vi "压装试验判定.vi"(7 "Result":refnum<vi>, 10 "判定参数":T1, 11 "XY曲线":cluster{"X":dbl[], "Y":dbl[]}[](array[cluster])) -> (2 "判定项长度":i32, 3 "OK？":bool)   [LabVIEW 2020]
panel:
  out "上限":dbl
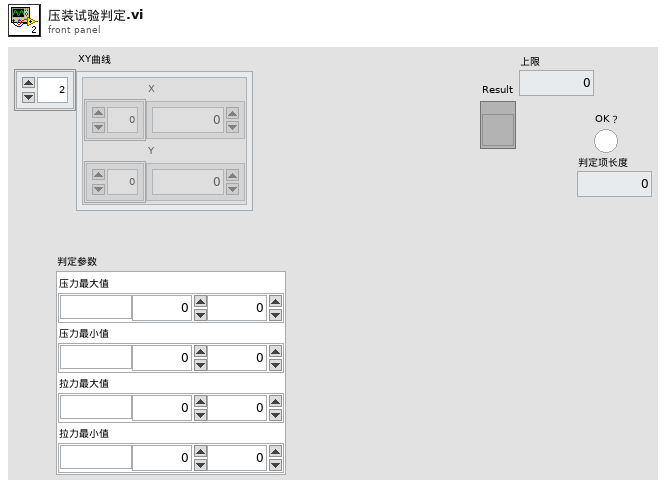
[diagram p1: front panel]
types:
  T1 = cluster{"压力最大值":cluster{"单位":string, "下限":dbl, "上限":dbl}, "压力最小值":cluster{"单位":string, "下限":dbl, "上限":dbl}, "拉力最大值":cluster{"单位":string, "下限":dbl, "上限":dbl}, "拉力最小值":cluster{"单位":string, "下限":dbl, "上限":dbl}}
  T2 = cluster{"位移":cluster{"单位":string, "下限":dbl, "上限":dbl}, "压力":cluster{"单位":string, "下限":dbl, "上限":dbl}}
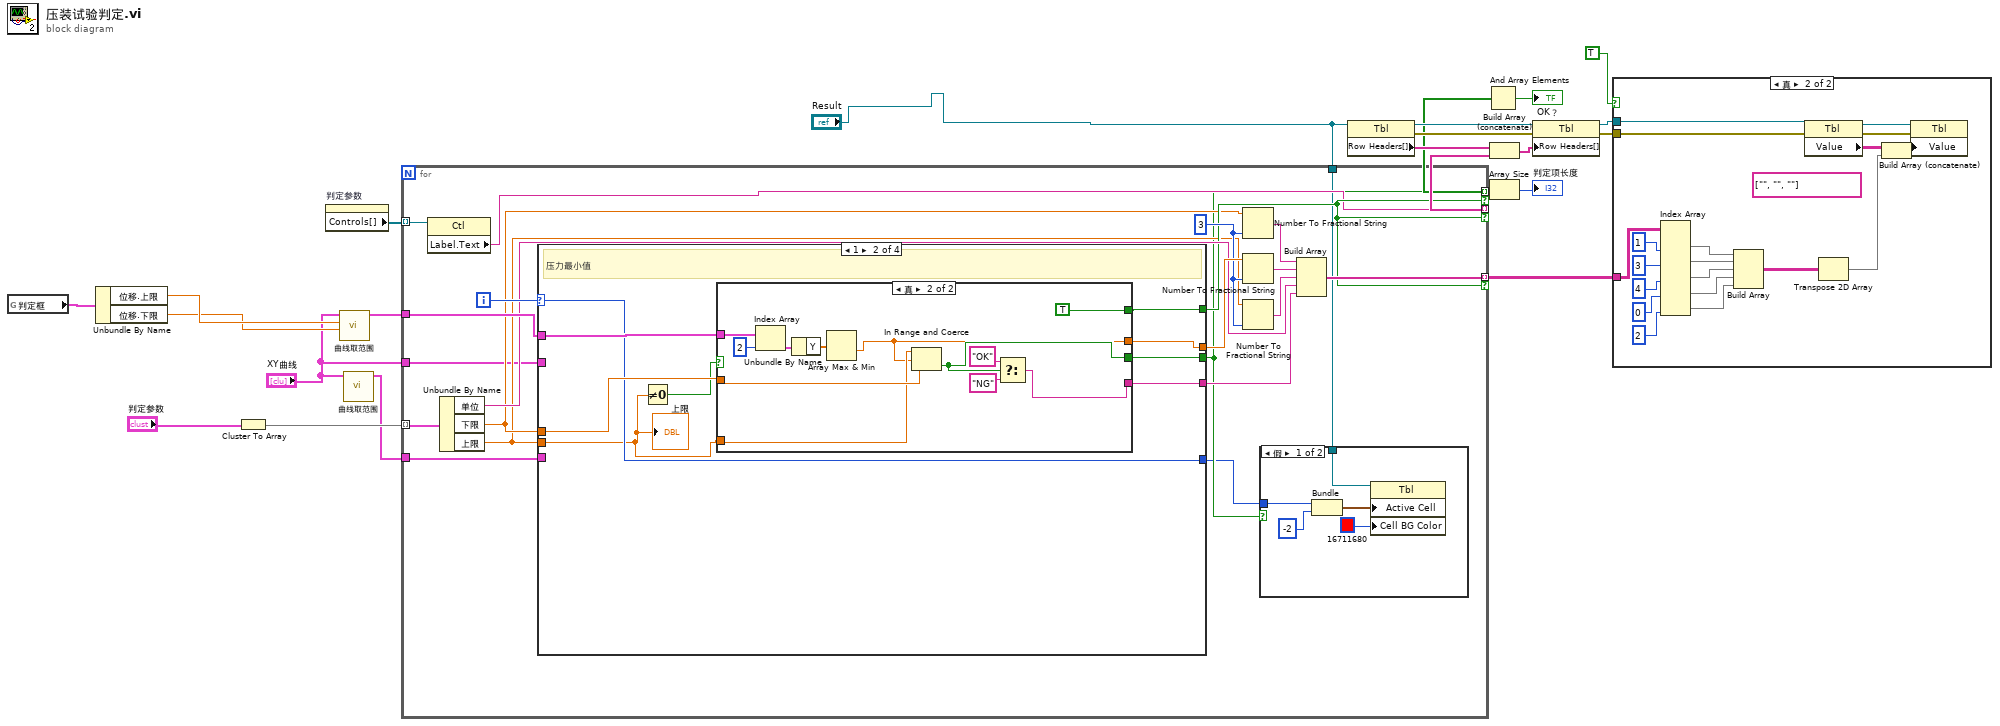
[diagram p0: block diagram]
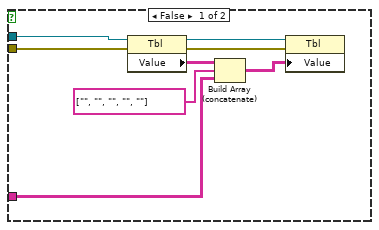
[diagram p2: hidden frame]
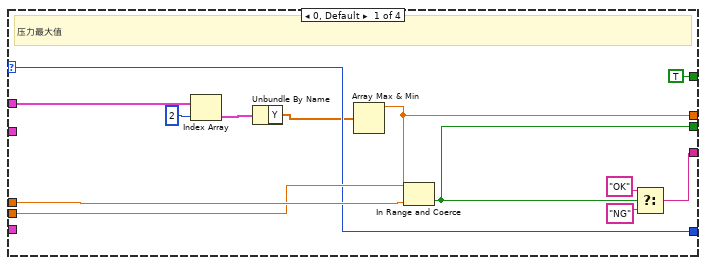
[diagram p4: hidden frame]
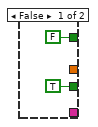
[diagram p5: hidden frame]
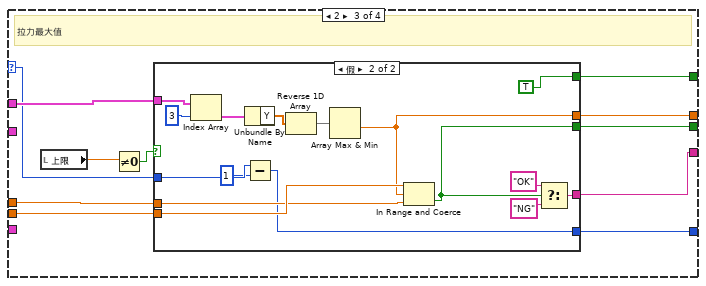
[diagram p6: hidden frame]
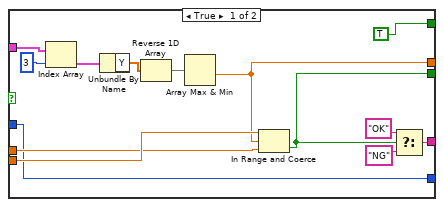
[diagram p7: hidden frame]
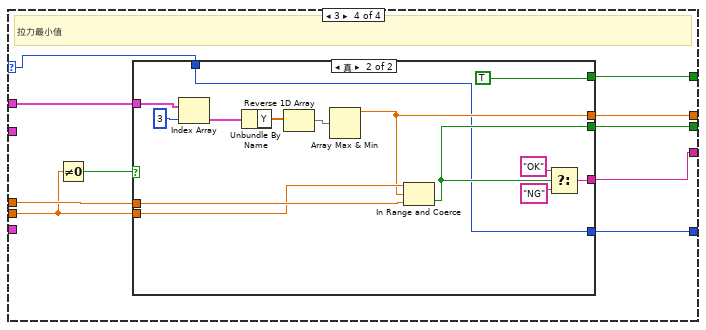
[diagram p8: hidden frame]
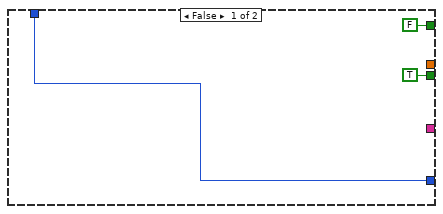
[diagram p9: hidden frame]
diagram:
  n1 = global read "判定参数.vi" "判定框"() -> (w4:T2)
  n2 = Unbundle By Name(w4) -> ("位移.上限"=w6:dbl, "位移.下限"=w5:dbl)
  n3 = Cluster To Array(cluster="判定参数") -> (array=w22:cluster{"单位":string, "下限":dbl, "上限":dbl}[])
  n4 = property on="判定参数" class="Clust (严格)"() -> ("Controls[]"=w12:refnum<vi>[])  [unwired: 2 in, 2 out]
  n5 = call "曲线取范围.vi"("下限"=w5, "上限"=w6, "曲线In"="XY曲线") -> ("曲线Out"=w8:cluster{"X":dbl[], "Y":dbl[]}[])  [unwired: 8 in]
  n6 = call "曲线取范围.vi"("曲线In"="XY曲线") -> ("曲线Out"=w2:cluster{"X":dbl[], "Y":dbl[]}[])  [unwired: 10 in]
  n7 = for {
    tunnel: w22 -> [w43] mode=indexing
    tunnel: w12 -> [w41] mode=indexing
    tunnel: w8 -> [w39]
    tunnel: [w24] -> w10 mode=indexing if=w31
    tunnel: [w32] -> w13 mode=indexing if=w31
    tunnel: [w28] -> w15 mode=indexing if=w31
    tunnel: "XY曲线" -> [w27]
    tunnel: w2 -> [w26]
    tunnel: "Result" -> [w25]
    i -> [w42]
    w38 = i16 3 ("精度(6)")
    n8 = property class="Ctl"(reference=w41) -> ("Label.Text"=w28:string)  [unwired: 1 in, 2 out]
    n9 = Unbundle By Name(w43) -> ("单位"=w33:string, "下限"=w30:dbl, "上限"=w29:dbl)
    n10 = case shown="1" w42 {
      selector: w42 -> [w51 w65 w86 w127]
      tunnel: [w49 w64 w92 w132] -> w40
      tunnel: w39 -> [w61 w70 w91 w131]
      tunnel: [w56 w69 w95 w135] -> w34
      tunnel: [w55 w68 w94 w134] -> w24
      tunnel: w30 -> [w54 w67 w90 w130]
      tunnel: w29 -> [w53 w62 w93 w128]
      tunnel: [TRUE w66 w89 w133] -> w31
      tunnel: w27 -> [_ _ _ _]
      tunnel: w26 -> [_ _ _ _]
      tunnel: [w51 w65 w85 w126] -> w23
      frame 0, Default {
        # "压力最大值"
        n11 = Index Array(array=w61, index=2 ("索引")) -> (element=w59:cluster{"X":dbl[], "Y":dbl[]})
        n12 = Unbundle By Name(w59) -> ("Y"=w50:dbl[])
        n13 = Array Max & Min(array=w50) -> (max value=w49:dbl)  [unwired: 3 out]
        n14 = In Range and Coerce(upper limit=w53, x=w49, lower limit=w54) -> (In Range?=w55:bool)  [unwired: 1 out]
        n15 = Select(t="OK", s=w55, f="NG") -> (s? t:f=w56:string)
      }
      frame 1 {
        # "压力最小值"
        n16 = Not Equal To 0?(x=w62) -> (x != 0?=w63:bool)
        n17 = case shown="真" w63 {
          tunnel: w70 -> [_ w84]
          tunnel: [_ w80] -> w69
          tunnel: [TRUE w79] -> w68
          tunnel: w67 -> [_ w78]
          tunnel: w62 -> [_ w77]
          tunnel: [FALSE TRUE] -> w66
          tunnel: [_ w73] -> w64
          frame False {
          }
          frame True {
            n18 = Index Array(array=w84, index=2 ("索引")) -> (element=w83:cluster{"X":dbl[], "Y":dbl[]})
            n19 = Unbundle By Name(w83) -> ("Y"=w75:dbl[])
            n20 = Array Max & Min(array=w75) -> (min value=w73:dbl)  [unwired: 3 out]
            n21 = In Range and Coerce(upper limit=w77, x=w73, lower limit=w78) -> (In Range?=w79:bool)  [unwired: 1 out]
            n22 = Select(t="OK", s=w79, f="NG") -> (s? t:f=w80:string)
          }
        }
        "上限" <- w62
      }
      frame 2 {
        # "拉力最大值"
        n23 = local read "上限"() -> (w87:dbl)
        n24 = Not Equal To 0?(x=w87) -> (x != 0?=w88:bool)
        n25 = case shown="假" w88 {
          tunnel: [w109 w125] -> w95
          tunnel: [w108 w124] -> w94
          tunnel: w93 -> [w107 w123]
          tunnel: [w106 w122] -> w92
          tunnel: w91 -> [w105 w121]
          tunnel: w90 -> [w104 w120]
          tunnel: [TRUE TRUE] -> w89
          tunnel: w86 -> [w96 w112]
          tunnel: [w96 w111] -> w85
          frame True {
            n26 = Index Array(array=w105, index=3 ("索引")) -> (element=w99:cluster{"X":dbl[], "Y":dbl[]})
            n27 = Unbundle By Name(w99) -> ("Y"=w98:dbl[])
            n28 = Reverse 1D Array(array=w98) -> (reversed array=w97:dbl[])
            n29 = Array Max & Min(array=w97) -> (min value=w106:dbl)  [unwired: 3 out]
            n30 = In Range and Coerce(upper limit=w107, x=w106, lower limit=w104) -> (In Range?=w108:bool)  [unwired: 1 out]
            n31 = Select(t="OK", s=w108, f="NG") -> (s? t:f=w109:string)
          }
          frame False {
            n32 = Index Array(array=w121, index=3 ("索引")) -> (element=w115:cluster{"X":dbl[], "Y":dbl[]})
            n33 = Unbundle By Name(w115) -> ("Y"=w114:dbl[])
            n34 = Subtract(x=w112, y=1) -> (x-y=w111:i32)
            n35 = Reverse 1D Array(array=w114) -> (reversed array=w113:dbl[])
            n36 = Array Max & Min(array=w113) -> (min value=w122:dbl)  [unwired: 3 out]
            n37 = In Range and Coerce(upper limit=w123, x=w122, lower limit=w120) -> (In Range?=w124:bool)  [unwired: 1 out]
            n38 = Select(t="OK", s=w124, f="NG") -> (s? t:f=w125:string)
          }
        }
      }
      frame 3 {
        # "拉力最小值"
        n39 = Not Equal To 0?(x=w128) -> (x != 0?=w129:bool)
        n40 = case shown="真" w129 {
          tunnel: [_ w149] -> w135
          tunnel: [TRUE w148] -> w134
          tunnel: w130 -> [_ w147]
          tunnel: w128 -> [_ w146]
          tunnel: [FALSE TRUE] -> w133
          tunnel: [_ w140] -> w132
          tunnel: w131 -> [_ w142]
          tunnel: w127 -> [w136 w139]
          tunnel: [w136 w139] -> w126
          frame False {
          }
          frame True {
            n41 = Index Array(array=w142, index=3 ("索引")) -> (element=w144:cluster{"X":dbl[], "Y":dbl[]})
            n42 = Unbundle By Name(w144) -> ("Y"=w143:dbl[])
            n43 = Reverse 1D Array(array=w143) -> (reversed array=w141:dbl[])
            n44 = Array Max & Min(array=w141) -> (max value=w140:dbl)  [unwired: 3 out]
            n45 = In Range and Coerce(upper limit=w146, x=w140, lower limit=w147) -> (In Range?=w148:bool)  [unwired: 1 out]
            n46 = Select(t="OK", s=w148, f="NG") -> (s? t:f=w149:string)
          }
        }
      }
    }
    n47 = Number To Fractional String(number=w30, precision (6)=w38) -> (F-format string=w37:string)  [unwired: 2 in]
    n48 = Number To Fractional String(number=w40, precision (6)=w38) -> (F-format string=w36:string)  [unwired: 2 in]
    n49 = Number To Fractional String(number=w29, precision (6)=w38) -> (F-format string=w35:string)  [unwired: 2 in]
    n50 = case shown="假" w24 {
      tunnel: w25 -> [w48 _]
      tunnel: w23 -> [w44 _]
      frame False {
        n51 = Bundle(w44, "索引"=-2) -> (w45:cluster{i32, "索引":i32})  [unwired: 1 in]
        n52 = property class="Tbl"(reference=w48, "Active Cell"=w45, "Cell BG Color"=u32 16711680 ("活动单元格:单元格背景色")) -> ()  [unwired: 1 in, 2 out]
      }
      frame True {
      }
    }
    n53 = Build Array(w37, w36, w35, w33, w34) -> (w32:string[])
  }
  n54 = property class="Tbl"(reference="Result") -> (reference out=w17:refnum<vi>, error out=w20:errorcluster, "Row Headers[]"=w14:string[])  [unwired: 1 in]
  n55 = And Array Elements(Boolean array=w10) -> (logical AND=→"OK？":bool)
  n56 = Build Array (concatenate)(w14, w15) -> (w16:string[])
  n57 = Array Size(array=w10) -> (size(s)=→"判定项长度":i32)
  n58 = property class="Tbl"(reference=w17, error in=w20, "Row Headers[]"=w16) -> (reference out=w18:refnum<vi>, error out=w19:errorcluster)
  n59 = case shown="真" TRUE {
    tunnel: w19 -> [w158 w177]
    tunnel: w18 -> [w155 w174]
    tunnel: w13 -> [w154 w173]
    frame False {
      n60 = property class="Tbl"(reference=w155, error in=w158) -> (reference out=w156:refnum<vi>, error out=w157:errorcluster, "Value"=w159:string[][])
      n61 = Build Array (concatenate)(w159, string[] ["", "", "", "", ""], w154) -> (w160:string[][])
      n62 = property class="Tbl"(reference=w156, error in=w157, "Value"=w160) -> ()  [unwired: 2 out]
    }
    frame True {
      (unwired) string[] ["", "", ""]
      n63 = Index Array(array=w173, index (col) #1=1 ("禁用的索引 (列)"), index (col) #2=3 ("索引 (列)"), index (col) #3=4 ("索引 (列)"), index (col) #4=0 ("索引 (列)"), index (col) #5=2 ("索引 (列)")) -> (element #1=w169:string[], element #2=w168:string[], element #3=w167:string[], element #4=w162:string[], element #5=w161:string[])  [unwired: 5 in]
      n64 = Build Array(w169, w168, w167, w162, w161) -> (w166:string[][])
      n65 = property class="Tbl"(reference=w174, error in=w177) -> (reference out=w175:refnum<vi>, error out=w176:errorcluster, "Value"=w178:string[][])
      n66 = Transpose 2D Array(2D array=w166) -> (transposed array=w165:string[][])
      n67 = Build Array (concatenate)(w178, w165) -> (w179:string[][])
      n68 = property class="Tbl"(reference=w175, error in=w176, "Value"=w179) -> ()  [unwired: 2 out]
    }
  }
